vi "Write_Normalize.vi"(9 "Normalized Data":dbl[][](array[numeric]), 10 "seconds since 1Jan1904":timestamp, 11 "Nornamiled":path=path "C:/Users/Chris/Desktop/DCS(Upgrade)/dcs_data/dcs_normalized.csv") -> ()   [LabVIEW 2013]
uses:
  <vilib>/Utility/file.llb/Write To Spreadsheet File (DBL).vi
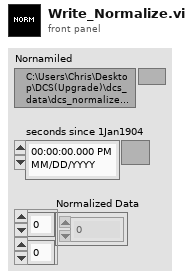
[diagram p1: front panel]
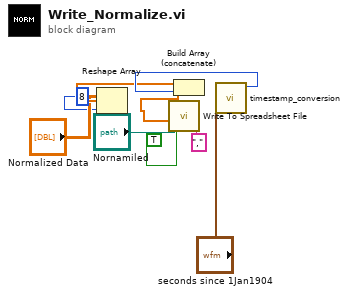
[diagram p0: block diagram]
diagram:
  n1 = Reshape Array("Normalized Data", 8 ("dimension size")) -> (w6:dbl[])
  n2 = call "timestamp_conversion.vi"("Time Stamp"="seconds since 1Jan1904") -> ("Integer Time"=w8:i64)  [unwired: 8 in, 1 out]
  n3 = Build Array (concatenate)(w6, w8) -> (w7:dbl[])
  n4 = call-poly <vilib>:"Write To Spreadsheet File.vi"("delimiter (\\t)"="," ("delimiter (\\t)"), "append to file? (new file:F)"=TRUE, "1D data"=w7, "file path (dialog if empty)"="Nornamiled") -> ()  [unwired: 4 in, 1 out]
